vi "Buffer_flushBuffer.vi"(8 "error in (no error)":errorcluster, 11 "Multiplexer_Opmux in":refnum<class "Multiplexer_Opmux.lvclass">) -> (0 "error out":errorcluster, 3 "Multiplexer_Opmux out":refnum<class "Multiplexer_Opmux.lvclass">)   [LabVIEW 2014, in "Multiplexer_Opmux.lvclass"]
uses:
  Multiplexer_Opmux.lvclass
  Multiplexer_Opmux.lvclass/Multiplexer_Opmux.ctl
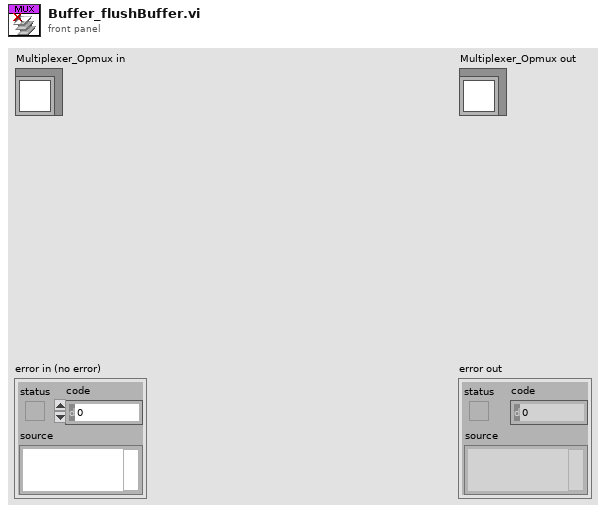
[diagram p1: front panel]
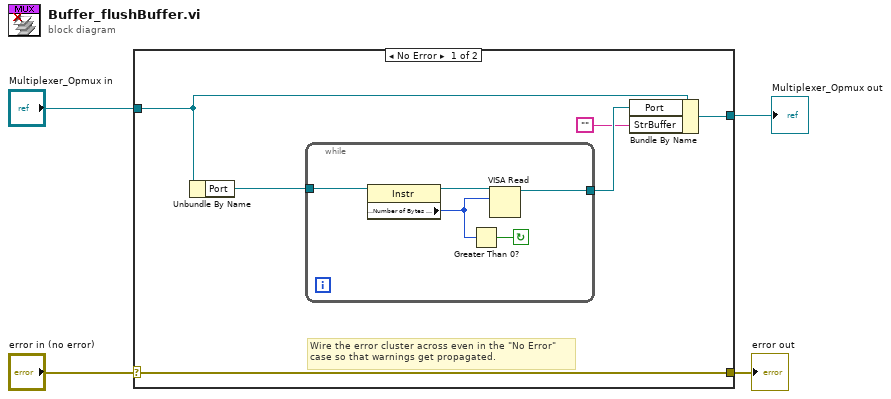
[diagram p0: block diagram]
diagram:
  n1 = case shown="No Error" "error in (no error)" {
    selector: "error in (no error)" -> [w10 w17]
    tunnel: [w10 w17] -> w3
    tunnel: [w7 w16] -> w1
    tunnel: "Multiplexer_Opmux in" -> [w8 w16]
    frame No Error {
      # "Wire the error cluster across even in the \"No Error\"\ncase so that warnings get propagated."
      n2 = Unbundle By Name(w8) -> ("Port"=w9:refnum<visa-resource-name>)
      n3 = while {
        tunnel: w9 -> [w12]
        tunnel: [w11] -> w6
        stop <- w13 continue-if-true
        n4 = property class="Instr"(reference=w12) -> (reference out=w15:refnum<visa-resource-name>, "Serial Settings:Number of Bytes at Serial Port"=w14:u32)  [unwired: 1 in, 1 out]
        n5 = Greater Than 0?(x=w14) -> (x > 0?=w13:bool)
        n6 = VISA Read(VISA resource name=w15, byte count=w14) -> (VISA resource name out=w11:refnum<visa-resource-name>)  [unwired: 1 in, 3 out]
      }
      n7 = Bundle By Name(cluster=w8, "Port"=w6, "StrBuffer"="") -> (w7:refnum<class "Multiplexer_Opmux.lvclass">)
    }
    frame Error {
    }
  }
  "error out" <- w3
  "Multiplexer_Opmux out" <- w1
